vi "Read to Buffer.vi"(8 "error in":errorcluster, 11 "Messaging Manager Actor in":refnum<class "Messaging Manager Actor.lvclass">) -> (0 "error out":errorcluster, 3 "Messaging Manager Actor out":refnum<class "Messaging Manager Actor.lvclass">)   [LabVIEW 2024, in "PCAN.lvlib" / "Messaging Manager Actor.lvlib" / "Messaging Manager Actor.lvclass"]
uses:
  Messaging Manager Actor.lvclass
  Messaging Manager Actor.lvclass/Messaging Manager Actor.ctl
  CAN Message/CAN Message.lvclass
  Messaging Buffer/Message Buffer.lvclass
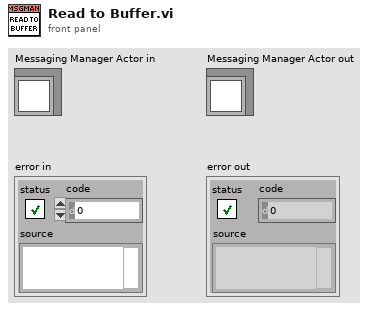
[diagram p1: front panel]
types:
  T1 = typedef "TPCANHandle.ctl" = enum16{"PCAN_NONEBUS  0x000", "PCAN_ISABUS1  0x21", "PCAN_ISABUS2  0x22", "PCAN_ISABUS3  0x23", "PCAN_ISABUS4  0x24", "PCAN_ISABUS5  0x25", "PCAN_ISABUS6  0x26", "PCAN_ISABUS7  0x27", "PCAN_ISABUS8  0x28", "PCAN_DNGBUS1  0x31", "PCAN_PCIBUS1  0x41", "PCAN_PCIBUS1  0x42", "PCAN_PCIBUS1  0x43", "PCAN_PCIBUS1  0x44", "PCAN_PCIBUS1  0x45", "PCAN_PCIBUS1  0x46", "PCAN_PCIBUS1  0x47", "PCAN_PCIBUS1  0x48", "PCAN_PCIBUS1  0x409", "PCAN_PCIBUS1  0x40A", "PCAN_PCIBUS1  0x40B", "PCAN_PCIBUS1  0x40C", "PCAN_PCIBUS1  0x40D", "PCAN_PCIBUS1  0x40E", "PCAN_PCIBUS1  0x40F", "PCAN_PCIBUS1  0x410", "PCAN_USBBUS1  0x51", "PCAN_USBBUS2  0x52", "PCAN_USBBUS3  0x53", "PCAN_USBBUS4  0x54", "PCAN_USBBUS5  0x55", "PCAN_USBBUS6  0x56", "PCAN_USBBUS7  0x57", "PCAN_USBBUS8  0x58", "PCAN_USBBUS9  0x509", "PCAN_USBBUS10  0x50A", "PCAN_USBBUS11  0x50B", "PCAN_USBBUS12  0x50C", "PCAN_USBBUS13  0x50D", "PCAN_USBBUS14  0x50E", "PCAN_USBBUS15  0x50F", "PCAN_USBBUS16  0x510", "PCAN_PCCBUS1  0x61", "PCAN_PCCBUS2  0x62", "PCAN_LANBUS1  0x801", "PCAN_LANBUS2  0x802", "PCAN_LANBUS3  0x803", "PCAN_LANBUS4  0x804", "PCAN_LANBUS5  0x805", "PCAN_LANBUS6  0x806", "PCAN_LANBUS7  0x807", "PCAN_LANBUS8  0x808", "PCAN_LANBUS9  0x809", "PCAN_LANBUS10  0x80A", "PCAN_LANBUS11  0x80B", "PCAN_LANBUS12  0x80C", "PCAN_LANBUS13  0x80D", "PCAN_LANBUS14  0x80E", "PCAN_LANBUS15  0x80F", "PCAN_LANBUS16  0x810"}
  T2 = typedef "TPCANTimestamp.ctl" = cluster{"millis overflow":u16, "millis ":u32, "micros":u16}
  T3 = typedef "CAN MSG Cluster.ctl" = cluster{"ID":u32, "MSG type":u8, "DLC":u8, "DATA":u8[]}
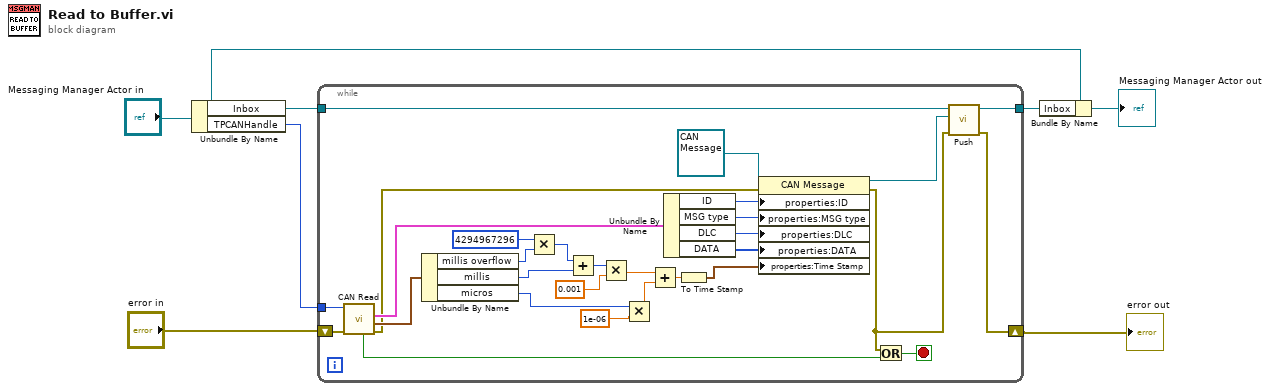
[diagram p0: block diagram]
diagram:
  n1 = Unbundle By Name("Messaging Manager Actor in") -> ("Inbox"=w6:refnum<class "Message Buffer.lvclass">, "TPCANHandle"=w7:T1)
  n2 = while {
    tunnel: w7 -> [w34]
    shift-right: [w9] -> w2
    shift-left: "error in" -> [w33]
    tunnel: w6 -> [w12]
    tunnel: [w8] -> w5
    stop <- w14 stop-if-true
    n3 = call <instrlib>:"CAN Read.vi"("error in (no error)"=w33, "TPCANHandle"=w34) -> ("error out"=w15:errorcluster, "TPCANTimestamp out"=w36:T2, "CAN_Message out"=w35:T3, "rcv queue empty"=w13:bool)  [unwired: 5 in, 1 out]
    n4 = Unbundle By Name(w36) -> ("millis overflow"=w24:u16, "millis"=w27:u32, "micros"=w26:u16)
    n5 = Multiply(x=u64 4294967296, y=w24) -> (x*y=w22:u64)
    n6 = Add(x=w22, y=w27) -> (x+y=w23:u64)
    n7 = Multiply(x=w23, y=0.001) -> (x*y=w29:dbl)
    n8 = Multiply(x=w26, y=1e-06) -> (x*y=w30:dbl)
    n9 = Add(x=w29, y=w30) -> (x+y=w28:dbl)
    n10 = Unbundle By Name(w35) -> ("ID"=w16:u32, "MSG type"=w17:u8, "DLC"=w18:u8, "DATA"=w19:u8[])
    n11 = To Time Stamp(1:w28) -> (0:w20:timestamp)
    n12 = property class="CAN Message"(reference=refnum<class "CAN Message.lvclass"> refnum ("PCAN.lvlib:Message.lvclass"), error in=w15, "properties:ID"=w16, "properties:MSG type"=w17, "properties:DLC"=w18, "properties:DATA"=w19, "properties:Time Stamp"=w20) -> (reference out=w11:refnum<class "CAN Message.lvclass">, error out=w10:errorcluster)
    n13 = Or(x=w10, y=w13) -> (x .or. y?=w14:bool)
    n14 = call "Push.vi"("error in"=w10, "IMessage"=w11, "Message Buffer in"=w12) -> ("error out"=w9:errorcluster, "Message Buffer out"=w8:refnum<class "Message Buffer.lvclass">)  [unwired: 7 in]
  }
  "error out" <- w2
  n15 = Bundle By Name(cluster="Messaging Manager Actor in", "Inbox"=w5) -> (→"Messaging Manager Actor out":refnum<class "Messaging Manager Actor.lvclass">)
